vi "One Hot.vi"(1 "hot index":u64, 2 "length":u64) -> (0 "One hot vector":T1)   [LabVIEW 2014]
uses:
  <vilib>/Analysis/Matrix/Datatypes/RealMatrix.ctl
  <vilib>/Analysis/Matrix/NI_Matrix.lvlib
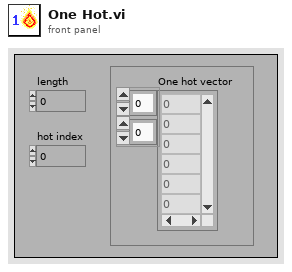
[diagram p1: front panel]
types:
  T1 = typedef "NI_Matrix.lvlib/RealMatrix.ctl" = dbl[][]
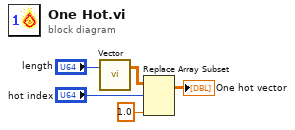
[diagram p0: block diagram]
diagram:
  n1 = call "Vector.vi"("length"="length") -> ("Real Matrix (Column Vector)"=w4:T1)  [unwired: 18 in]
  n2 = Replace Array Subset(array=w4, new element=1.0 ("new element/submatrix"), index (row)="hot index") -> (→"One hot vector":T1)  [unwired: 1 in]
